vi "Create FIFO.vi"(8 "error in (no error)":errorcluster, 9 "FIFO Name":string, 10 "TX?":bool, 11 "Comm FIFOs Virtual Folder":refnum<vi>) -> (0 "error out":errorcluster, 3 "Comm FIFOs Virtual Folder":refnum<vi>)   [LabVIEW 2014, in "Initialization and IO Node Scripting.lvlib"]
uses:
  Initialization and IO Node Scripting.lvlib
  <vilib>/rvi/ClientSDK/Core/Script/Fifo/ProjectItem/Public/nirviPiFifoType_Size.ctl
  <vilib>/rvi/ClientSDK/Core/Script/Fifo/ProjectItem/Private/nirviPiFifo_OpenWithProjectItem.vi
  <vilib>/rvi/ClientSDK/Core/Script/Fifo/ProjectItem/Private/nirviPiFifo_SetDataType2.vi
  <vilib>/rvi/ClientSDK/Core/Script/Fifo/ProjectItem/Private/nirviPiFifo_SetSize.vi
  <vilib>/rvi/ClientSDK/Core/Script/Fifo/ProjectItem/Private/nirviPiFifo_CommitGlobal.vi
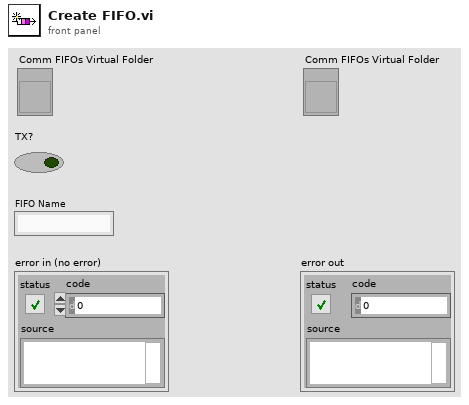
[diagram p1: front panel]
types:
  T1 = typedef "nirviPiFifoType_Size.ctl" = u32
  T2 = cluster{"Device ID":u8, "Data":u64, "Command":u8, "Node ID":u8, "Misc":u8}
  T3 = typedef "nirviPiFifo_State.ctl" = cluster{"Item":refnum<vi>, "Fifo":T4, "Dirty":bool, "XNode":refnum<vi>}
  T4 = typedef "niFpgaContainerState.ctl" = cluster{"displayName":string, "hardwareName":string, "dataType":T5, "elementTypeDescriptor":variant, "terminalTypeDescriptor":variant, "requestedNumberOfElements":u32, "memoryType":T6, "arbitrationForInterfaceA":T7, "numberOfElementsPerRead":u32, "arbitrationForInterfaceB":T7, "numberOfElementsPerWrite":u32, "VI_Defined":bool, "type":T8, "initializationParameters":T9, "disableOnOverflow/Underflow":bool, "interfaceConfiguration":T10, "controlLogic":T11, "actualNumberOfElements":u32, "dramSelection":string, "dramMaxOustandingRequests":i32, "dramIncludeByteEnables":bool, "dramGrantTime":u32, "fullEmulation":bool, "memoryInMultipleClockDomains":bool, "memoryLatency":T12}
  T5 = typedef "niFpgaDataTypeControl.ctl" = enum32{"Boolean", "I8", "I16", "I32", "I64", "U8", "U16", "U32", "U64", "FXP", "CustomControl", "SGL"}
  T6 = typedef "niFpgaContainerImplementationControl.ctl" = enum16{"Flip-Flops", "Look-Up Table", "Block Memory", "DRAM"}
  T7 = typedef "niFpgaContainerArbitrationOptionsControl.ctl" = enum16{"Always Arbitrate", "Arbitrate if Multiple Requestors Only", "Never Arbitrate"}
  T8 = typedef "niFpgaTransferTypeControl.ctl" = enum16{"Target-Scoped", "Host to Target - DMA", "Target to Host - DMA", "Peer to Peer Reader", "Peer to Peer Writer", "Bidirectional"}
  T9 = typedef "niFpgaContainerInitializationParameters.ctl" = cluster{"initialized":bool, "VI_Path":path, "initialData":variant}
  T10 = typedef "niFpgaMemoryInterfaceConfiguration.ctl" = enum16{"Read A-Write B", "Read A-Read B"}
  T11 = typedef "niFpgaFifoControlLogicControl.ctl" = enum16{"Slice Fabric", "Target Optimal", "Built-in"}
  T12 = typedef "niFpgaContainerMemoryLatencyControl.ctl" = u16
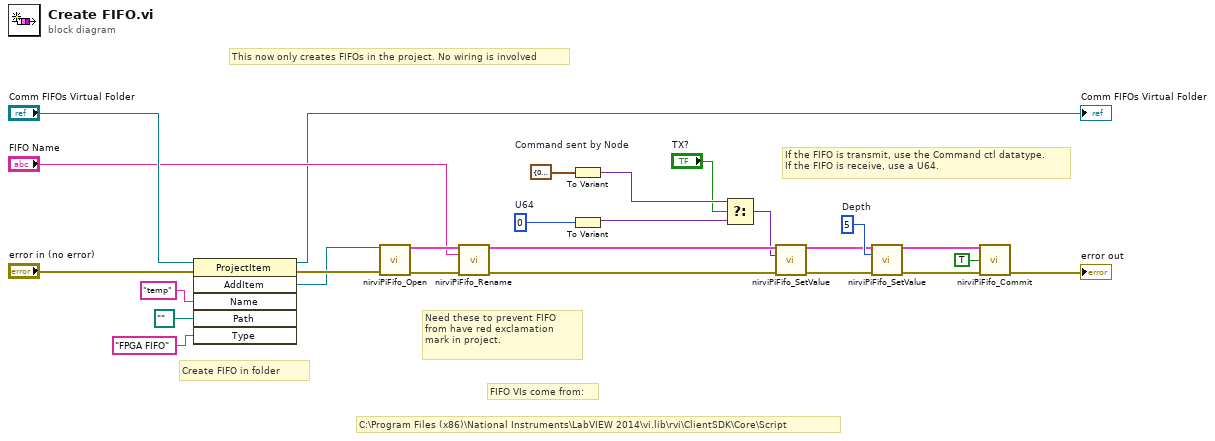
[diagram p0: block diagram]
diagram:
  w5 = T1 5  # Depth
  w10 = u64 0  # U64
  w11 = T2 {"Device ID"=0, "Data"=0, "Command"=0, "Node ID"=0, "Misc"=0}  # Command sent by Node
  # "If the FIFO is transmit, use the Command ctl datatype.\nIf the FIFO is receive, use a U64."
  # "FIFO VIs come from:"
  # "This now only creates FIFOs in the project. No wiring is involved"
  # "Create FIFO in folder"
  # "Need these to prevent FIFO from have red exclamation mark in project."
  # "C:\\Program Files (x86)\\National Instruments\\LabVIEW 2014\\vi.lib\\rvi\\ClientSDK\\Core\\Script"
  n1 = invoke class="ProjectItem" method="AddItem"(reference="Comm FIFOs Virtual Folder", error in="error in (no error)", "Name"="temp", "Path"=path "", "Type"="FPGA FIFO") -> (reference out=→"Comm FIFOs Virtual Folder":refnum<vi>, error out=w18:errorcluster, "AddItem"=w15:refnum<vi>)  [unwired: 1 in, 3 out]
  n2 = call-poly <vilib>:"nirviPiFifo_Open.vi"("Fifo Item"=w15, "error in (no error)"=w18) -> ("Reference"=w25:T3, "error out"=w26:errorcluster)  [unwired: 12 in]
  n3 = call <vilib>:"nirviPiFifo_Rename.vi"("reference"=w25, "name"="FIFO Name", "error in (no error)"=w26) -> ("reference"=w13:T3, "error out"=w12:errorcluster)  [unwired: 11 in]
  n4 = To Variant(anything=w11) -> (Variant=w9:variant)
  n5 = To Variant(anything=w10) -> (Variant=w7:variant)
  n6 = Select(t=w9, s="TX?", f=w7) -> (s? t:f=w6:variant)
  n7 = call-poly "nirviPiFifo_SetValue.vi"("Reference"=w13, "Data Type"=w6, "error in (no error)"=w12) -> ("Reference"=w1:T3, "error out"=w4:errorcluster)  [unwired: 11 in]
  n8 = call-poly "nirviPiFifo_SetValue.vi"("Reference"=w1, "Size"=w5, "error in (no error)"=w4) -> ("Reference"=w2:T3, "error out"=w3:errorcluster)  [unwired: 11 in]
  n9 = call-poly <vilib>:"nirviPiFifo_Commit.vi"("Reference"=w2, "Close Reference?"=TRUE, "error in (no error)"=w3) -> ("error out"=→"error out":errorcluster)  [unwired: 11 in, 1 out]
